vi "JKISM++ Send Message and Wait for Reply.vi"(6 "Response Timeout(1000ms)":i32=10000, 8 "Error In (no error)":errorcluster, 9 "Dest Module":string="A", 10 "Arguments (\"\")":string, 11 "States":string="DoA") -> (0 "error IO":errorcluster, 2 "Arguments":string="DoA")   [LabVIEW 2014, in "JKI-State-Machine-Plus.lvlib"]
uses:
  JKI-State-Machine-Plus.lvlib
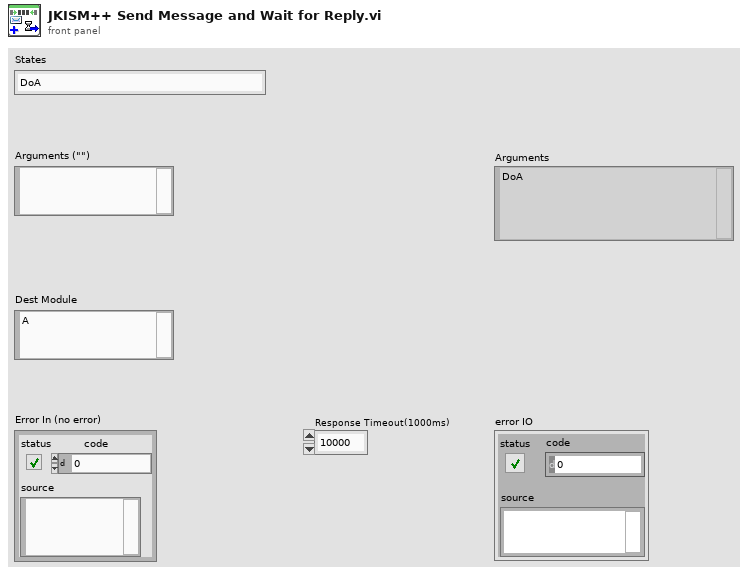
[diagram p1: front panel]
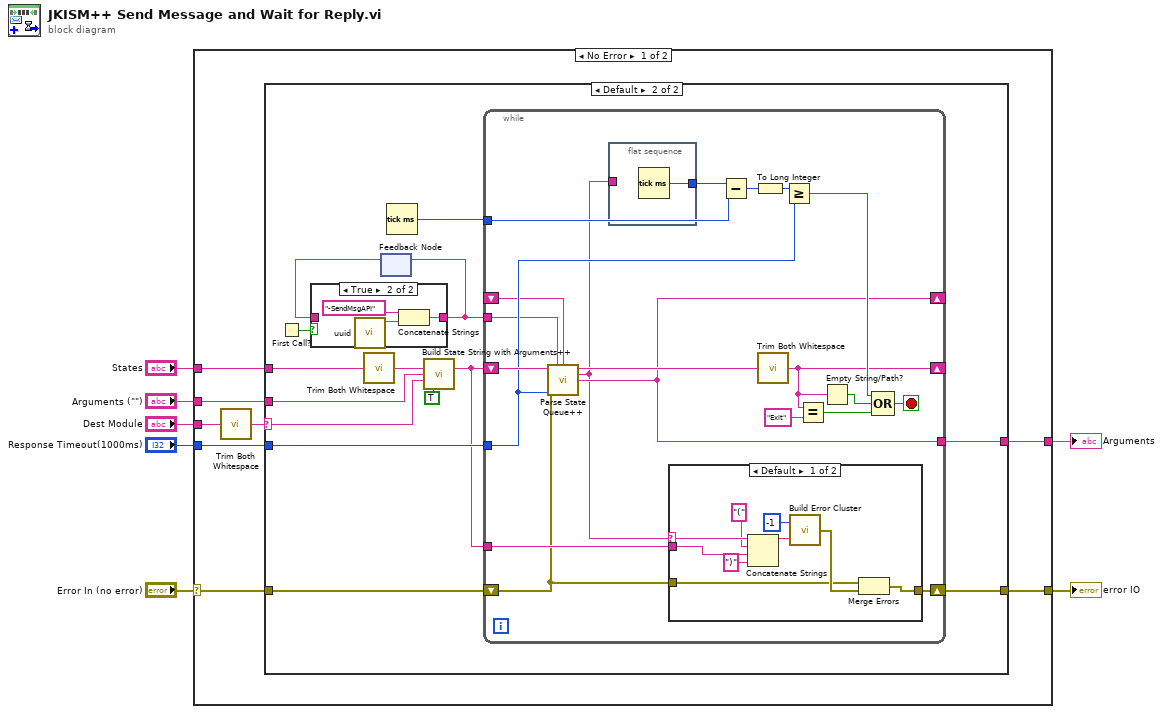
[diagram p0: block diagram]
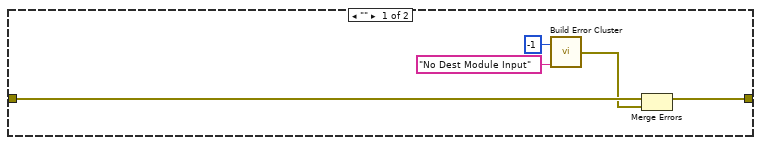
[diagram p2: hidden frame]
diagram:
  n1 = case shown="No Error" "Error In (no error)" {
    selector: "Error In (no error)" -> [w14 w70]
    tunnel: "States" -> [w15 _]
    tunnel: "Response Timeout(1000ms)" -> [w13 _]
    tunnel: [w9 w70] -> w4
    tunnel: [w12 _] -> w3
    tunnel: "Dest Module" -> [w11 _]
    tunnel: "Arguments (\"\")" -> [w10 _]
    frame No Error {
      n2 = call "Trim Both Whitespace.vi"("string"=w11) -> ("trimmed string"=w8:string)  [unwired: 1 in]
      n3 = case shown="Default" w8 {
        selector: w8 -> [_ w27]
        tunnel: w15 -> [_ w34]
        tunnel: w14 -> [w18 w33]
        tunnel: w13 -> [_ w32]
        tunnel: [_ w30] -> w12
        tunnel: w10 -> [_ w26]
        tunnel: [w17 w25] -> w9
        frame "" {
          n4 = call "Build Error Cluster.vi"("String to Prepend to source (\"\")"="No Dest Module Input" ("String to Prepend to source (\"\")"), "code"=-1) -> ("error out"=w16:errorcluster)
          n5 = Merge Errors(w18, w16) -> (w17:errorcluster)
        }
        frame Default {
          n6 = First Call?() -> (First Call?: T/F=w22:bool)
          n7 = call "Trim Both Whitespace.vi"("string"=w34) -> ("trimmed string"=w28:string)  [unwired: 1 in]
          n8 = feedback #1() -> (w21:string)  [unwired: 1 in]
          n9 = case shown="True" w22 {
            tunnel: [w35 w36] -> w23
            tunnel: w21 -> [w35 _]
            frame False {
            }
            frame True {
              n10 = call "uuid.vi"() -> ("UUID"=w37:string)  [unwired: 11 in]
              n11 = Concatenate Strings("-SendMsgAPI" ("Name(\"\" to use uuid)"), w37) -> (w36:string)
            }
          }
          n12 = feedback-in #1(w23) -> ()
          n13 = Tick Count (ms)() -> (millisecond timer value=w31:u32)
          n14 = call "Build State String with Arguments++.vi"("State"=w28, "Arguments (\"\")"=w26, "Dest Module (\"\")"=w27, "Sync-Call(@) T By Default/Async-Call(->) F"=TRUE) -> ("State with Arguments"=w24:string)  [unwired: 11 in]
          n15 = while {
            shift-right: [w39] -> _
            shift-left: w24 -> [w58]
            tunnel: w32 -> [w52]
            tunnel: w31 -> [w55]
            tunnel: [w49] -> w30
            shift-right: [w49] -> _
            shift-left: _ -> [w48]
            tunnel: w23 -> [w47]
            tunnel: w24 -> [w45]
            shift-right: [w44] -> w25
            shift-left: w33 -> [w43]
            stop <- w54 stop-if-true
            n16 = call "Parse State Queue++.vi"("State Queue"=w58, "Name(\"\" to use uuid)"=w47, "Response Arguments"=w48, "Error In (no error)"=w43, "Response Timeout(5000ms)"=w52) -> ("Remaining States"=w57:string, "Current State"=w46:string, "Arguments"=w49:string)  [unwired: 5 in, 3 out]
            n17 = flat-sequence {
              tunnel: [w69] -> w56
              tunnel: w46 -> [_]
              frame #0 {
                n18 = Tick Count (ms)() -> (millisecond timer value=w69:u32)
              }
            }
            n19 = case shown="Default" w46 {
              selector: w46 -> [w66 _]
              tunnel: [w63 w68] -> w44
              tunnel: w43 -> [w62 w68]
              tunnel: w45 -> [w61 _]
              frame Default {
                n20 = Concatenate Strings(w66, "(" ("string"), w61, ")" ("string")) -> (w65:string)
                n21 = call "Build Error Cluster.vi"("String to Prepend to source (\"\")"=w65, "code"=-1) -> ("error out"=w64:errorcluster)
                n22 = Merge Errors(w62, w64) -> (w63:errorcluster)
              }
              frame "Response" {
              }
            }
            n23 = Subtract(x=w56, y=w55) -> (x-y=w53:u32)
            n24 = To Long Integer(number=w53) -> (32bit integer=w50:i32)
            n25 = call "Trim Both Whitespace.vi"("string"=w57) -> ("trimmed string"=w39:string)  [unwired: 1 in]
            n26 = Greater Or Equal?(x=w50, y=w52) -> (x >= y?=w51:bool)
            n27 = Equal?(x=w39, y="Exit" ("State(s) at Back (\"\")")) -> (x = y?=w42:bool)
            n28 = Empty String/Path?(string/path=w39) -> (empty?=w40:bool)
            n29 = Compound Arithmetic op=OR(w51, w40, w42) -> (w54:bool)
          }
        }
      }
    }
    frame Error {
    }
  }
  "error IO" <- w4
  "Arguments" <- w3
